vi "Get Root Path.vi"(11 "VI in":refnum<vi>) -> (3 "Extpad Directory":path)   [LabVIEW 2025, in "Interface Functions.lvlib"]
uses:
  Interface Functions.lvlib
  <vilib>/Utility/LVLibp/NI_PackedLibraryUtility.lvlib
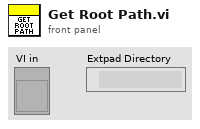
[diagram p1: front panel]
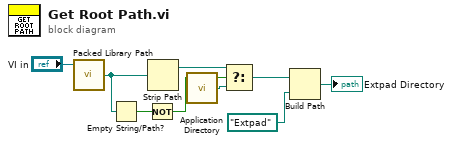
[diagram p0: block diagram]
diagram:
  n1 = call <vilib>:"Packed Library Path.vi"("vi reference"="VI in") -> ("packed library path"=w7:path)  [unwired: 2 in, 2 out]
  n2 = Empty String/Path?(string/path=w7) -> (empty?=w8:bool)
  n3 = Not(x=w8) -> (.not. x?=w9:bool)
  n4 = Strip Path(path=w7) -> (stripped path=w5:path)  [unwired: 1 out]
  n5 = call <vilib>:"Application Directory.vi"() -> ("Application Directory"=w6:path)
  n6 = Select(t=w5, s=w9, f=w6) -> (s? t:f=w3:path)
  n7 = Build Path(base path=w3, name or relative path=path "Extpad") -> (appended path=→"Extpad Directory":path)
